vi "Create.vi"(8 "error in (no error)":errorcluster, 11 "GrabberTool Class in":refnum<class "GrabberTool Class.lvclass">) -> (0 "error out":errorcluster, 3 "GrabberTool Class out":refnum<class "GrabberTool Class.lvclass">)   [LabVIEW 2011, in "GrabberTool Class.lvclass"]
uses:
  GrabberTool Class.lvclass
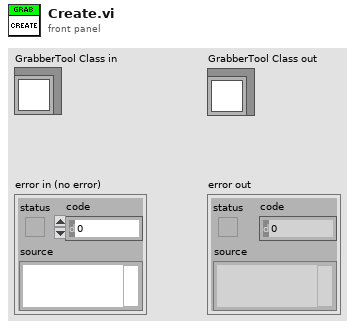
[diagram p1: front panel]
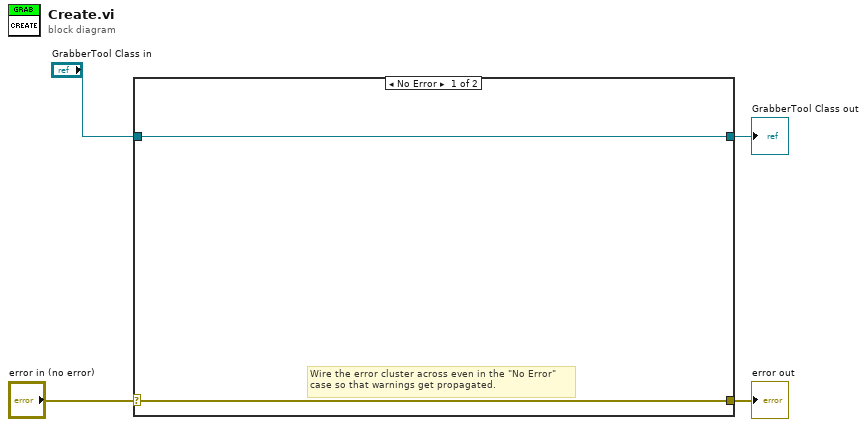
[diagram p0: block diagram]
diagram:
  n1 = case shown="No Error" "error in (no error)" {
    selector: "error in (no error)" -> [w5 w8]
    tunnel: [w5 w8] -> w3
    tunnel: [w6 w7] -> w1
    tunnel: "GrabberTool Class in" -> [w6 w7]
    frame No Error {
      # "Wire the error cluster across even in the \"No Error\"\ncase so that warnings get propagated."
    }
    frame Error {
    }
  }
  "error out" <- w3
  "GrabberTool Class out" <- w1
